vi "ADIS16470 IMU Example New.vi"() -> ()   [LabVIEW 2018]
uses:
  <vilib>/Utility/RT CPU Load.ctl
  ADIS16470Lib/Typedef/ADIS16470 Hardware Configuration.ctl
  <vilib>/Rock Robotics/WPI/SPI/WPI_SPIMode.ctl
  <vilib>/Rock Robotics/SystemInterfaces/DIO/FPGA_DIOChannel.ctl
  <vilib>/Rock Robotics/SystemInterfaces/spilib/spi_bus.ctl
  <vilib>/NI_Real-Time Target Support.lvlib
panel:
  out "Ready?":bool
  in  "Hardware Config":T1={"SPI Clock Rate (Hz)"=2000000.0, "IMU SPI Mode (3)"=enum."Mode 3 (Clk Idle High,Sample on Trailing)", "IMU Reset Pin"=enum."SPI Port CS2", "IMU SPI Bus"=enum."SPI On-Board, CS0", "IMU Data Ready Pin"=enum."SPI Port CS1"}
  out "CPU loads":T5[](array[typedef]) {"ISR (%)" format="%#.2f"; "Idle (%)" format="%#.2f"; "Background (%)" format="%#.2f"; "Normal (%)" format="%#.2f"; "Above Normal (%)" format="%#.2f"; "High (%)" format="%#.2g"; "Timed Structures (%)" format="%#.2g"; "Time Critical (%)" format="%#.2g"; "Total (%)" format="%#.2g"}
  in  "stop":bool
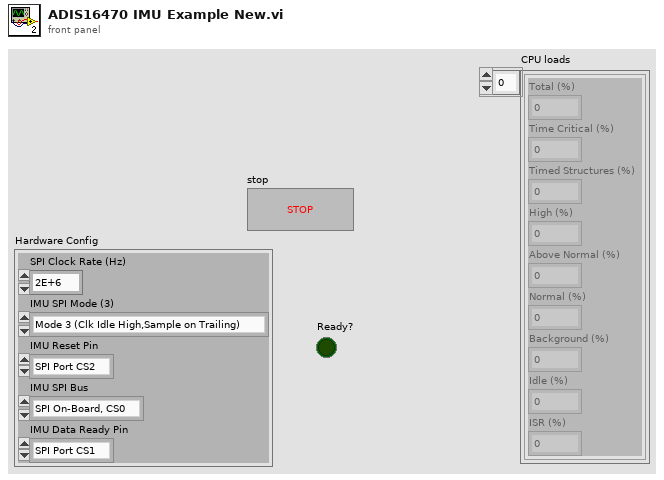
[diagram p1: front panel]
types:
  T1 = typedef "ADIS16470 Hardware Configuration.ctl" = cluster{"SPI Clock Rate (Hz)":dbl, "IMU SPI Mode (3)":T2, "IMU Reset Pin":T3, "IMU SPI Bus":T4, "IMU Data Ready Pin":T3}
  T2 = typedef "WPI_SPIMode.ctl" = enum16{"Mode 0 (Clk Idle Low,Sample on Leading)", "Mode 1 (Clk Idle Low,Sample on Trailing)", "Mode 2 (Clk Idle High,Sample on Leading)", "Mode 3 (Clk Idle High,Sample on Trailing)"}
  T3 = typedef "FPGA_DIOChannel.ctl" = enum8{"DIO 0", "DIO 1", "DIO 2", "DIO 3", "DIO 4", "DIO 5", "DIO 6", "DIO 7", "DIO 8", "DIO 9", "DIO MXP 0", "DIO MXP 1", "DIO MXP 2", "DIO MXP 3", "DIO MXP 4", "DIO MXP 5", "DIO MXP 6", "DIO MXP 7", "DIO MXP 8", "DIO MXP 9", "DIO MXP 10", "DIO MXP 11", "DIO MXP 12", "DIO MXP 13", "DIO MXP 14", "DIO MXP 15", "SPI Port CS1", "SPI Port CS2", "SPI Port CS3", "SPI Port MISO", "SPI Port MOSI", "Invalid"}
  T4 = typedef "spi_bus.ctl" = enum16{"SPI On-Board, CS0", "SPI On-Board, CS1", "SPI On-Board, CS2", "SPI On-Board, CS3", "SPI MXP", "Invalid"}
  T5 = typedef "NI_Real-Time Target Support.lvlib/RT CPU Load.ctl" = cluster{"Total (%)":dbl, "Time Critical (%)":dbl, "Timed Structures (%)":dbl, "High (%)":dbl, "Above Normal (%)":dbl, "Normal (%)":dbl, "Background (%)":dbl, "Idle (%)":dbl, "ISR (%)":dbl}
  T6 = typedef "ADIS16470 Device Reference.ctl" = cluster{"DevStatus":errorcluster, "Hardware Config":T1, "End Calibration":refnum<k4>, "Calibration Complete":refnum<k4>}
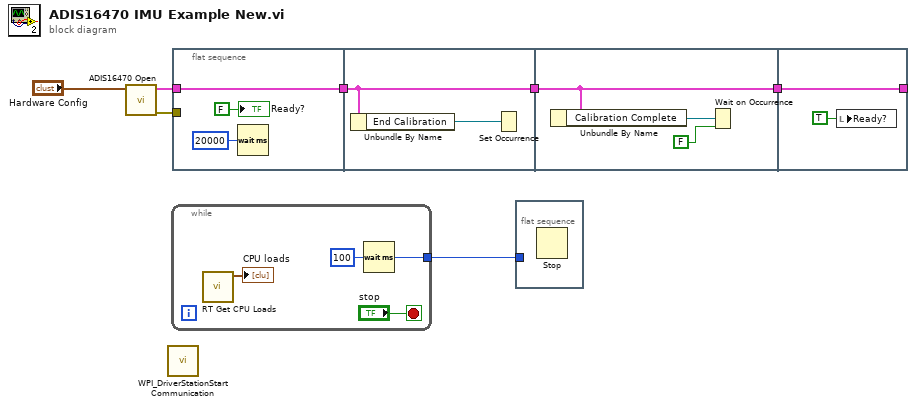
[diagram p0: block diagram]
diagram:
  n1 = call "ADIS16470 Open.vi"("Hardware Config"="Hardware Config") -> ("error out"=w4:errorcluster, "ADIS16470DevRef"=w5:T6)  [unwired: 9 in]
  n2 = call <vilib>:"WPI_DriverStationStart Communication.vi"() -> ()  [unwired: 12 in]
  n3 = while {
    tunnel: [w8] -> w7
    stop <- "stop" stop-if-true
    n4 = call <vilib>:"RT Get CPU Loads.vi"() -> ("CPU loads"=→"CPU loads":T5[])  [unwired: 10 in, 1 out]
    n5 = Wait (ms)(milliseconds to wait=u32 100) -> (millisecond timer value=w8:u32)
  }
  n6 = flat-sequence {
    tunnel: w5 -> [w13]
    tunnel: w4 -> [_]
    tunnel: [w13] -> w3
    tunnel: w3 -> [w15]
    tunnel: [w15] -> w2
    tunnel: w2 -> [w19]
    tunnel: [w19] -> w1
    tunnel: [w21] -> _
    tunnel: w1 -> [w21]
    frame #0 {
      n7 = Wait (ms)(milliseconds to wait=u32 20000) -> ()  [unwired: 1 out]
      "Ready?" <- FALSE ("Ready?")
    }
    frame #1 {
      n8 = Unbundle By Name(w15) -> ("End Calibration"=w16:refnum<k4>)
      n9 = Set Occurrence(w16) -> ()
    }
    frame #2 {
      n10 = Unbundle By Name(w19) -> ("Calibration Complete"=w18:refnum<k4>)
      n11 = Wait on Occurrence(1:FALSE ("ignore previous (T)"), 2:w18) -> ()  [unwired: 1 in, 1 out]
    }
    frame #3 {
      n12 = local write "Ready?"(TRUE ("Ready?")) -> ()
    }
  }
  n13 = flat-sequence {
    tunnel: w7 -> [_]
    frame #0 {
      n14 = Stop() -> ()  [unwired: 1 in]
    }
  }
